vi "Main.vi"() -> ()   [LabVIEW 2022 SP3]
uses:
  StateENUM.ctl
  1d93126f-b57a-4b2e-a5e1-2b10a66ae46b.vi
  <vilib>/Instr/_visa.llb/VISA Configure Serial Port (Instr).vi
panel:
  in  "stop 3":bool
  out "Waveform Chart":dbl(graph)
  in  "VISA resource name 2":refnum<visa-resource-name>
  in  "Check Center":bool
  out "Step":i32
  in  "Increase Step":bool
  in  "Decrease Step":bool
  out "Center":i32
  out "LoopCount":i32
  in  "Jitter Up":bool
  in  "Jitter Down":bool
  out "Command Buffer":string
  in  "stop":bool
  out "Current Time":timestamp format="%<%I:%M:%S %p | %m/%d/%y>T"
  in  "VISA resource name":refnum<visa-resource-name>="COM9"
  in  "Up Button":bool
  in  "Down Button":bool
  # "Manual\nAdjustment"
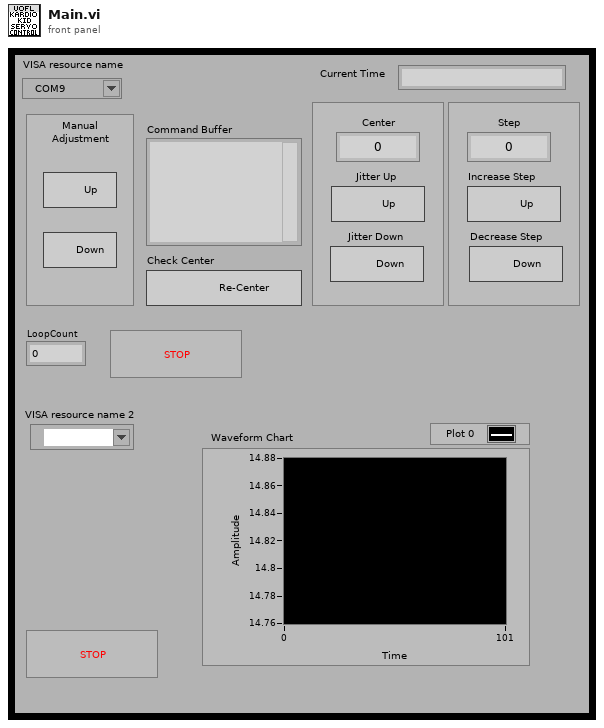
[diagram p1: front panel]
types:
  T1 = typedef "StateENUM.ctl" = enum16{"Init", "Idle", "MoveUp", "MoveDown", "JitterUp", "JitterDown", "IncreaseStep", "DecreaseStep", "CheckCenter", "ReadSerial", "ScanData", "Shutdown"}
  T2 = cluster{"VISA resource name out":refnum<visa-resource-name>, "error out":errorcluster, "State":T1, "Stop":bool, "Buffer":string, "Center":i32, "Step":i32, "SerialIncoming?":bool}
  T3 = cluster{"Command Buffer":refnum<vi>, "Jitter Up":refnum<vi>, "Jitter Down":refnum<vi>, "Increase Step":refnum<vi>, "Decrease Step":refnum<vi>}
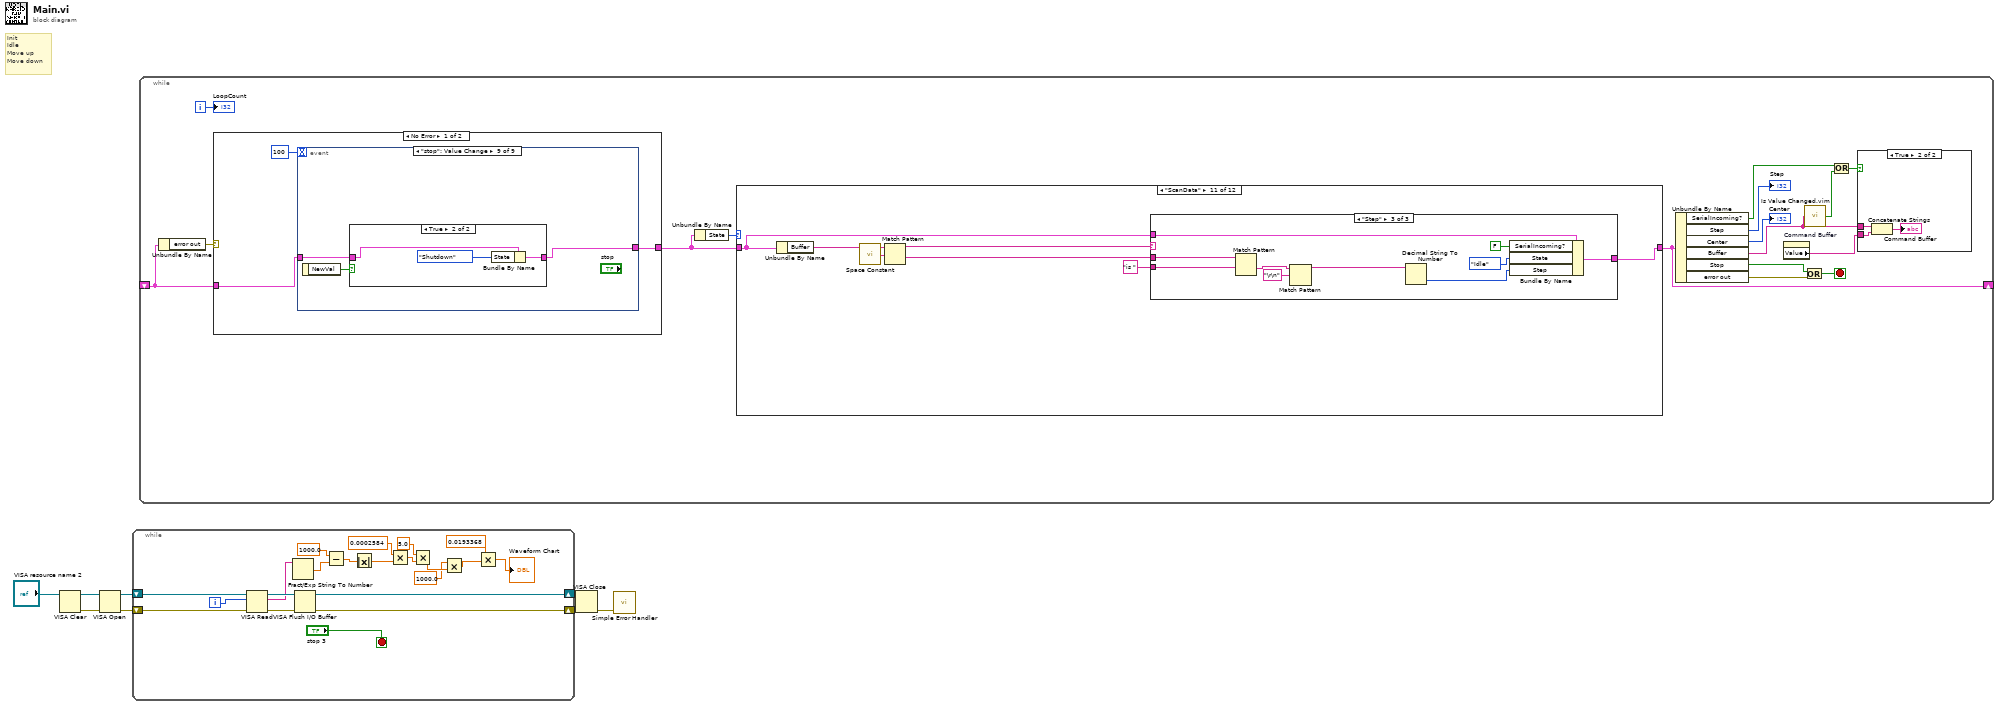
[diagram p0: block diagram]
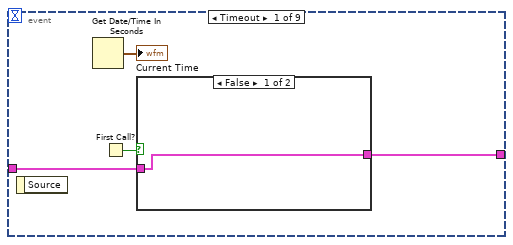
[diagram p3: hidden frame]
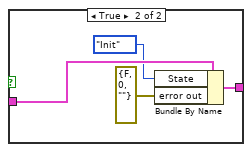
[diagram p4: hidden frame]
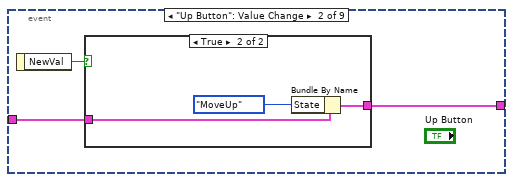
[diagram p5: hidden frame]
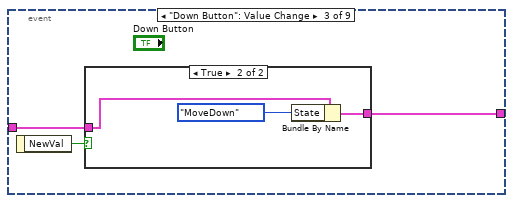
[diagram p7: hidden frame]
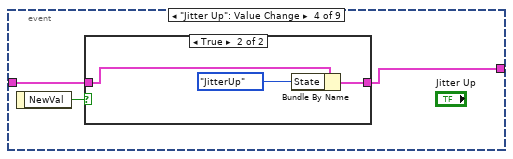
[diagram p9: hidden frame]
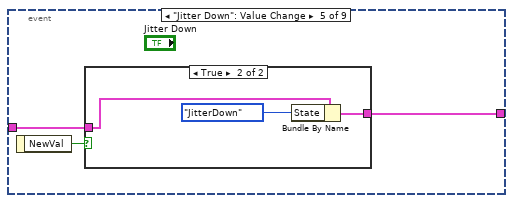
[diagram p11: hidden frame]
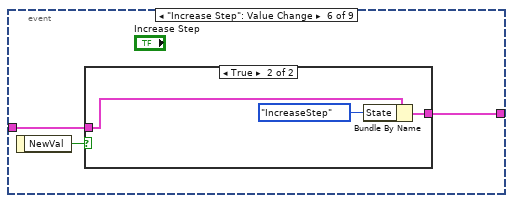
[diagram p13: hidden frame]
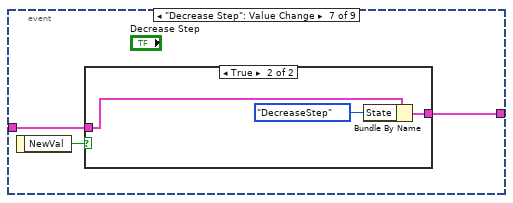
[diagram p15: hidden frame]
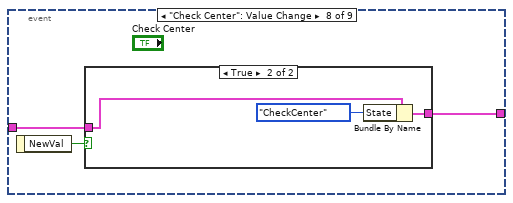
[diagram p17: hidden frame]
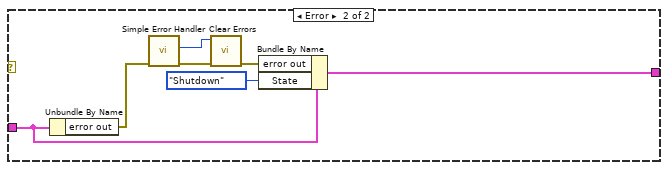
[diagram p20: hidden frame]
diagram:
  # "Init\nIdle\nMove up\nMove down"
  n1 = VISA Clear(VISA resource name="VISA resource name 2") -> (VISA resource name out=w5:refnum<visa-resource-name>, error out=w6:errorcluster)  [unwired: 1 in]
  n2 = VISA Open(error in (no error)=w6, VISA resource name=w5) -> (VISA resource name=w1:refnum<visa-resource-name>, error out=w2:errorcluster)  [unwired: 3 in]
  n3 = while {
    shift-right: [w26] -> w4
    shift-left: w1 -> [w29]
    shift-right: [w27] -> w3
    shift-left: w2 -> [w28]
    i -> [w22]
    stop <- "stop 3" stop-if-true
    n4 = VISA Read(VISA resource name=w29, byte count=w22, error in (no error)=w28) -> (VISA resource name out=w25:refnum<visa-resource-name>, read buffer=w23:string, error out=w24:errorcluster)  [unwired: 1 out]
    n5 = Fract/Exp String To Number(string=w23) -> (number=w20:dbl)  [unwired: 3 in, 1 out]
    n6 = VISA Flush I/O Buffer(VISA resource name=w25, error in (no error)=w24) -> (VISA resource name out=w26:refnum<visa-resource-name>, error out=w27:errorcluster)  [unwired: 1 in]
    n7 = Subtract(x=1000.0, y=w20) -> (x-y=w18:dbl)
    n8 = Absolute Value(x=w18) -> (abs(x)=w17:dbl)
    n9 = Multiply(x=0.0002584, y=w17) -> (x*y=w15:dbl)
    n10 = Multiply(x=5.0, y=w15) -> (x*y=w10:dbl)
    n11 = Multiply(x=1000.0, y=w10) -> (x*y=w11:dbl)
    n12 = Multiply(x=0.0193368, y=w11) -> (x*y=→"Waveform Chart":dbl)
  }
  n13 = while {
    shift-right: [w43] -> _
    shift-left: _ -> [w42]
    i -> [w30]
    stop <- w39 stop-if-true
    n14 = Unbundle By Name(w42) -> ("error out"=w41:errorcluster)
    n15 = case shown="No Error" w41 {
      tunnel: w42 -> [w50 w123]
      tunnel: [w49 w119] -> w44
      frame No Error {
        n16 = event shown="[8] \"stop\": Value Change" {
          selector: _ -> [_ _ _ _ _ _ _ _ _]
          dyn-events: _ -> [_ _ _ _ _ _ _ _ _]
          timeout: 100 -> [_ _ _ _ _ _ _ _ _]
          tunnel: w50 -> [w52 w63 w69 w77 w84 w91 w98 w105 w111]
          tunnel: [w53 w61 w68 w75 w82 w89 w96 w103 w110] -> w49
          event Timeout {
            n17 = event-data() -> ()  [unwired: 1 in, 1 out]
            n18 = Get Date/Time In Seconds() -> (seconds since 1Jan1904=→"Current Time":timestamp)
            n19 = First Call?() -> (First Call?: T/F=w54:bool)
            n20 = case shown="False" w54 {
              tunnel: [w56 w59] -> w53
              tunnel: w52 -> [w56 w60]
              frame False {
              }
              frame True {
                n21 = Bundle By Name(cluster=w60, "State"=StateENUM."Init", "error out"=errorcluster {"status"=FALSE, "code"=0, "source"=""}) -> (w59:T2)
              }
            }
          }
          event "Up Button": Value Change {
            n22 = event-data() -> ("NewVal"=w62:bool)  [unwired: 1 in]
            n23 = case shown="True" w62 {
              tunnel: w63 -> [w64 w67]
              tunnel: [w64 w66] -> w61
              frame False {
              }
              frame True {
                n24 = Bundle By Name(cluster=w67, "State"=StateENUM."MoveUp") -> (w66:T2)
              }
            }
          }
          event "Down Button": Value Change {
            n25 = event-data() -> ("NewVal"=w70:bool)  [unwired: 1 in]
            n26 = case shown="True" w70 {
              tunnel: w69 -> [w71 w74]
              tunnel: [w71 w73] -> w68
              frame False {
              }
              frame True {
                n27 = Bundle By Name(cluster=w74, "State"=StateENUM."MoveDown") -> (w73:T2)
              }
            }
          }
          event "Jitter Up": Value Change {
            n28 = event-data() -> ("NewVal"=w76:bool)  [unwired: 1 in]
            n29 = case shown="True" w76 {
              tunnel: w77 -> [w78 w81]
              tunnel: [w78 w80] -> w75
              frame False {
              }
              frame True {
                n30 = Bundle By Name(cluster=w81, "State"=StateENUM."JitterUp") -> (w80:T2)
              }
            }
          }
          event "Jitter Down": Value Change {
            n31 = event-data() -> ("NewVal"=w83:bool)  [unwired: 1 in]
            n32 = case shown="True" w83 {
              tunnel: w84 -> [w85 w88]
              tunnel: [w85 w87] -> w82
              frame False {
              }
              frame True {
                n33 = Bundle By Name(cluster=w88, "State"=StateENUM."JitterDown") -> (w87:T2)
              }
            }
          }
          event "Increase Step": Value Change {
            n34 = event-data() -> ("NewVal"=w90:bool)  [unwired: 1 in]
            n35 = case shown="True" w90 {
              tunnel: w91 -> [w92 w95]
              tunnel: [w92 w94] -> w89
              frame False {
              }
              frame True {
                n36 = Bundle By Name(cluster=w95, "State"=StateENUM."IncreaseStep") -> (w94:T2)
              }
            }
          }
          event "Decrease Step": Value Change {
            n37 = event-data() -> ("NewVal"=w97:bool)  [unwired: 1 in]
            n38 = case shown="True" w97 {
              tunnel: w98 -> [w99 w102]
              tunnel: [w99 w101] -> w96
              frame False {
              }
              frame True {
                n39 = Bundle By Name(cluster=w102, "State"=StateENUM."DecreaseStep") -> (w101:T2)
              }
            }
          }
          event "Check Center": Value Change {
            n40 = event-data() -> ("NewVal"=w104:bool)  [unwired: 1 in]
            n41 = case shown="True" w104 {
              tunnel: w105 -> [w106 w109]
              tunnel: [w106 w108] -> w103
              frame False {
              }
              frame True {
                n42 = Bundle By Name(cluster=w109, "State"=StateENUM."CheckCenter") -> (w108:T2)
              }
            }
          }
          event "stop": Value Change {
            n43 = event-data() -> ("NewVal"=w112:bool)  [unwired: 1 in]
            n44 = case shown="True" w112 {
              tunnel: w111 -> [w113 w116]
              tunnel: [w113 w115] -> w110
              frame False {
              }
              frame True {
                n45 = Bundle By Name(cluster=w116, "State"=StateENUM."Shutdown") -> (w115:T2)
              }
            }
          }
        }
      }
      frame Error {
        n46 = Unbundle By Name(w123) -> ("error out"=w122:errorcluster)
        n47 = call <vilib>:"Simple Error Handler.vi"("error in (no error)"=w122) -> ("code out"=w120:i32, "error out"=w121:errorcluster)  [unwired: 4 in, 3 out]
        n48 = call <vilib>:"Clear Errors.vi"("error in (no error)"=w121, "specific error code to clear (0: all)"=w120) -> ("error out"=w118:errorcluster)  [unwired: 4 in, 1 out]
        n49 = Bundle By Name(cluster=w123, "error out"=w118, "State"=StateENUM."Shutdown") -> (w119:T2)
      }
    }
    n50 = Unbundle By Name(w44) -> ("State"=w45:T1)
    n51 = case shown="\"ScanData\"" w45 {
      tunnel: [w142 w152 w158 w167 w178 w189 w198 w207 w216 w234 w251 w282] -> w43
      tunnel: w44 -> [_ w154 w159 w172 w183 w194 w203 w212 w221 w235 w252 w284]
      frame "Init", Default {
        w130 = FALSE  # SerialIncoming?
        w132 = 50  # Step
        w133 = 1500  # Center
        w135 = ""  # Buffer
        w140 = FALSE  # Stop
        w141 = StateENUM."Idle"  # State
        n52 = control-ref of="Command Buffer"() -> (w125:refnum<vi>)
        n53 = control-ref of="Decrease Step"() -> (w129:refnum<vi>)
        n54 = control-ref of="Increase Step"() -> (w128:refnum<vi>)
        n55 = control-ref of="Jitter Up"() -> (w126:refnum<vi>)
        n56 = control-ref of="Jitter Down"() -> (w127:refnum<vi>)
        n57 = Bundle("Command Buffer"=w125, "Jitter Up"=w126, "Jitter Down"=w127, "Increase Step"=w128, "Decrease Step"=w129) -> (w124:T3)  [unwired: 1 in]
        n58 = call "InitPostions (SubVI).vi"("ControlCluster"=w124) -> ()  [unwired: 11 in]
        n59 = Wait (ms)(milliseconds to wait=u32 5) -> ()  [unwired: 1 out]
        n60 = call-poly "VISA Configure Serial Port"("VISA resource name"="VISA resource name") -> ("VISA resource name out"=w138:refnum<visa-resource-name>, "error out"=w137:errorcluster)  [unwired: 13 in]
        n61 = VISA Flush I/O Buffer(VISA resource name=w138, error in (no error)=w137) -> (VISA resource name out=w131:refnum<visa-resource-name>, error out=w136:errorcluster)  [unwired: 1 in]
        n62 = Bundle("VISA resource name out"=w131, "error out"=w136, "State"=w141, "Stop"=w140, "Buffer"=w135, "Center"=w133, "Step"=w132, "SerialIncoming?"=w130) -> (w142:T2)  [unwired: 1 in]
      }
      frame "Idle" {
        n63 = Unbundle By Name(w154) -> ("State"=w145:T1, "VISA resource name out"=w151:refnum<visa-resource-name>, "error out"=w150:errorcluster)
        n64 = property class="Instr"(reference=w151, error in=w150) -> (error out=w149:errorcluster, "Serial Settings:Number of Bytes at Serial Port"=w147:u32)  [unwired: 1 out]
        n65 = Greater Than 0?(x=w147) -> (x > 0?=w144:bool)
        n66 = Select(t=StateENUM."ReadSerial" ("State"), s=w144, f=w145) -> (s? t:f=w148:T1)
        n67 = Bundle By Name(cluster=w154, "State"=w148, "error out"=w149, "SerialIncoming?"=FALSE) -> (w152:T2)
        n68 = Wait (ms)(milliseconds to wait=u32 5) -> ()  [unwired: 1 out]
      }
      frame "MoveUp" {
        n69 = Unbundle By Name(w159) -> ("VISA resource name out"=w163:refnum<visa-resource-name>, "error out"=w155:errorcluster)
        n70 = Concatenate Strings("0", "\r\n") -> (w160:string)
        n71 = VISA Write(VISA resource name=w163, write buffer=w160, error in (no error)=w155) -> (error out=w156:errorcluster)  [unwired: 2 out]
        n72 = Bundle By Name(cluster=w159, "State"=StateENUM."ReadSerial", "error out"=w156) -> (w158:T2)
      }
      frame "MoveDown" {
        # "49"
        n73 = Concatenate Strings("1", "\r\n") -> (w168:string)
        n74 = Unbundle By Name(w172) -> ("VISA resource name out"=w171:refnum<visa-resource-name>, "error out"=w164:errorcluster)
        n75 = VISA Write(VISA resource name=w171, write buffer=w168, error in (no error)=w164) -> (error out=w165:errorcluster)  [unwired: 2 out]
        n76 = Bundle By Name(cluster=w172, "State"=StateENUM."ReadSerial", "error out"=w165) -> (w167:T2)
      }
      frame "JitterUp" {
        n77 = Unbundle By Name(w183) -> ("Center"=w174:i32, "VISA resource name out"=w182:refnum<visa-resource-name>, "error out"=w175:errorcluster)
        n78 = Concatenate Strings("2", "\r\n") -> (w179:string)
        n79 = VISA Write(VISA resource name=w182, write buffer=w179, error in (no error)=w175) -> (error out=w176:errorcluster)  [unwired: 2 out]
        n80 = Increment(x=w174) -> (x+1=w173:i32)
        n81 = Bundle By Name(cluster=w183, "State"=StateENUM."ReadSerial", "Center"=w173, "error out"=w176) -> (w178:T2)
      }
      frame "JitterDown" {
        n82 = Unbundle By Name(w194) -> ("Center"=w185:i32, "VISA resource name out"=w193:refnum<visa-resource-name>, "error out"=w186:errorcluster)
        n83 = Concatenate Strings("3", "\r\n") -> (w190:string)
        n84 = VISA Write(VISA resource name=w193, write buffer=w190, error in (no error)=w186) -> (error out=w187:errorcluster)  [unwired: 2 out]
        n85 = Decrement(x=w185) -> (x-1=w184:i32)
        n86 = Bundle By Name(cluster=w194, "State"=StateENUM."ReadSerial", "Center"=w184, "error out"=w187) -> (w189:T2)
      }
      frame "IncreaseStep" {
        n87 = Unbundle By Name(w203) -> ("VISA resource name out"=w202:refnum<visa-resource-name>, "error out"=w195:errorcluster)
        n88 = Concatenate Strings("4", "\r\n") -> (w199:string)
        n89 = VISA Write(VISA resource name=w202, write buffer=w199, error in (no error)=w195) -> (error out=w196:errorcluster)  [unwired: 2 out]
        n90 = Bundle By Name(cluster=w203, "State"=StateENUM."ReadSerial", "error out"=w196) -> (w198:T2)
      }
      frame "DecreaseStep" {
        n91 = Unbundle By Name(w212) -> ("VISA resource name out"=w211:refnum<visa-resource-name>, "error out"=w204:errorcluster)
        n92 = Concatenate Strings("5", "\r\n") -> (w208:string)
        n93 = VISA Write(VISA resource name=w211, write buffer=w208, error in (no error)=w204) -> (error out=w205:errorcluster)  [unwired: 2 out]
        n94 = Bundle By Name(cluster=w212, "State"=StateENUM."ReadSerial", "error out"=w205) -> (w207:T2)
      }
      frame "CheckCenter" {
        n95 = Unbundle By Name(w221) -> ("VISA resource name out"=w220:refnum<visa-resource-name>, "error out"=w213:errorcluster)
        n96 = Concatenate Strings("6", "\r\n") -> (w217:string)
        n97 = VISA Write(VISA resource name=w220, write buffer=w217, error in (no error)=w213) -> (error out=w214:errorcluster)  [unwired: 2 out]
        n98 = Bundle By Name(cluster=w221, "State"=StateENUM."ReadSerial", "error out"=w214) -> (w216:T2)
      }
      frame "ReadSerial" {
        n99 = Unbundle By Name(w235) -> ("VISA resource name out"=w230:refnum<visa-resource-name>, "error out"=w225:errorcluster, "Buffer"=w224:string)
        n100 = property class="Instr"(reference=w230, error in=w225) -> (reference out=w227:refnum<visa-resource-name>, error out=w226:errorcluster, "Serial Settings:Number of Bytes at Serial Port"=w228:u32)
        n101 = Greater Than 0?(x=w228) -> (x > 0?=w229:bool)
        n102 = case shown="True" w229 {
          selector: w229 -> [w237 w241]
          tunnel: [w238 w246] -> w232
          tunnel: [w239 w245] -> w231
          tunnel: w226 -> [w239 w244]
          tunnel: w227 -> [_ w243]
          tunnel: w228 -> [_ w242]
          tunnel: w224 -> [w238 _]
          tunnel: [w237 w241] -> w223
          tunnel: [StateENUM."Idle" ("State") StateENUM."ScanData" ("State")] -> w222
          frame False {
          }
          frame True {
            n103 = VISA Read(VISA resource name=w243, byte count=w242, error in (no error)=w244) -> (read buffer=w246:string, error out=w245:errorcluster)  [unwired: 2 out]
          }
        }
        n104 = Bundle By Name(cluster=w235, "State"=w222, "SerialIncoming?"=w223, "Buffer"=w232, "error out"=w231) -> (w234:T2)
        n105 = Wait (ms)(milliseconds to wait=u32 5) -> ()  [unwired: 1 out]
      }
      frame "ScanData" {
        n106 = Unbundle By Name(w252) -> ("Buffer"=w253:string)
        n107 = call <vilib>:"Space Constant.vi"() -> ("String"=w248:string)
        n108 = Match Pattern(string=w253, regular expression=w248) -> (before substring=w247:string, after substring=w249:string)  [unwired: 1 in, 2 out]
        n109 = case shown="\"Step\"" w247 {
          tunnel: "is " -> [_ w267 w277]
          tunnel: w249 -> [_ w266 w276]
          tunnel: w252 -> [w257 w262 w272]
          tunnel: [w256 w260 w270] -> w251
          frame Default {
            n110 = Bundle By Name(cluster=w257, "State"=StateENUM."Idle", "SerialIncoming?"=FALSE) -> (w256:T2)
          }
          frame "Center", "Stop" {
            n111 = Match Pattern(string=w266, regular expression=w267) -> (after substring=w264:string)  [unwired: 1 in, 3 out]
            n112 = Match Pattern(string=w264, regular expression="\r\n") -> (before substring=w263:string)  [unwired: 1 in, 3 out]
            n113 = Decimal String To Number(string=w263) -> (number=w261:i32)  [unwired: 2 in, 1 out]
            n114 = Bundle By Name(cluster=w262, "SerialIncoming?"=FALSE, "State"=StateENUM."Idle", "Center"=w261) -> (w260:T2)
          }
          frame "Step" {
            n115 = Match Pattern(string=w276, regular expression=w277) -> (after substring=w274:string)  [unwired: 1 in, 3 out]
            n116 = Match Pattern(string=w274, regular expression="\r\n") -> (before substring=w273:string)  [unwired: 1 in, 3 out]
            n117 = Decimal String To Number(string=w273) -> (number=w271:i32)  [unwired: 2 in, 1 out]
            n118 = Bundle By Name(cluster=w272, "SerialIncoming?"=FALSE, "State"=StateENUM."Idle", "Step"=w271) -> (w270:T2)
          }
        }
      }
      frame "Shutdown" {
        n119 = Unbundle By Name(w284) -> ("VISA resource name out"=w283:refnum<visa-resource-name>, "error out"=w278:errorcluster)
        n120 = VISA Close(VISA resource name=w283, error in (no error)=w278) -> (error out=w279:errorcluster)
        n121 = Bundle By Name(cluster=w284, "Stop"=TRUE, "State"=StateENUM."Shutdown", "error out"=w279) -> (w282:T2)
      }
    }
    n122 = Unbundle By Name(w43) -> ("SerialIncoming?"=w32:bool, "Step"=→"Step":i32, "Center"=→"Center":i32, "Buffer"=w36:string, "Stop"=w38:bool, "error out"=w37:errorcluster)
    n123 = property on="Command Buffer" class="Str"() -> ("Value"=w35:string)  [unwired: 2 in, 2 out]
    n124 = Or(x=w38, y=w37) -> (x .or. y?=w39:bool)
    n125 = call "Is Value Changed.vim"("value"=w36) -> ("changed or first call?"=w34:bool)
    n126 = Or(x=w32, y=w34) -> (x .or. y?=w33:bool)
    n127 = case shown="True" w33 {
      tunnel: w36 -> [_ w48]
      tunnel: w35 -> [_ w47]
      frame False {
      }
      frame True {
        n128 = Concatenate Strings(w48, w47) -> (→"Command Buffer":string)
      }
    }
    "LoopCount" <- w30
  }
  n129 = VISA Close(VISA resource name=w4, error in (no error)=w3) -> (error out=w8:errorcluster)
  n130 = call <vilib>:"Simple Error Handler.vi"("error in (no error)"=w8) -> ()  [unwired: 4 in, 5 out]
